vi "TagCreatePixelArray.vi"(5 "Layout":string, 6 "Add Border":bool, 7 "Codes":i64[](array[numeric]), 8 "error in (no error)":errorcluster, 11 "ID":i32) -> (0 "error out":errorcluster, 1 "Alpha":u8[][](array[numeric]), 3 "Pixels":u8[][](array[numeric]))   [LabVIEW 2020, in "feature_detection.lvlib"]
uses:
  feature_detection.lvlib
  TagPixelType.ctl
  <vilib>/Utility/error.llb/Error Cluster From Error Code.vi
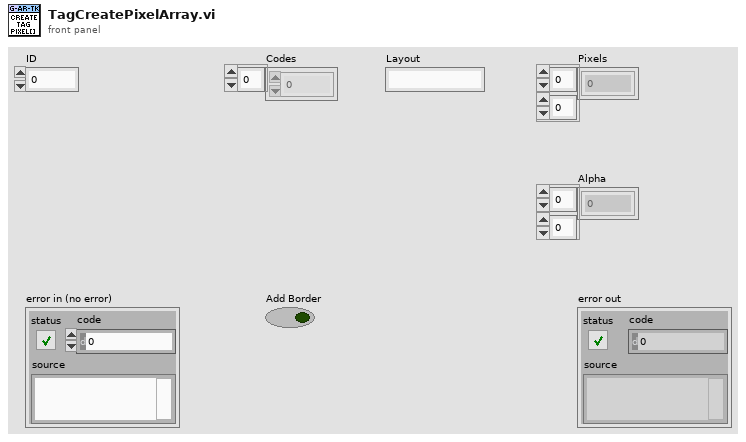
[diagram p1: front panel]
types:
  T1 = typedef "feature_detection.lvlib/TagPixelType.ctl" = enum8{"Black", "White", "Transparent"}
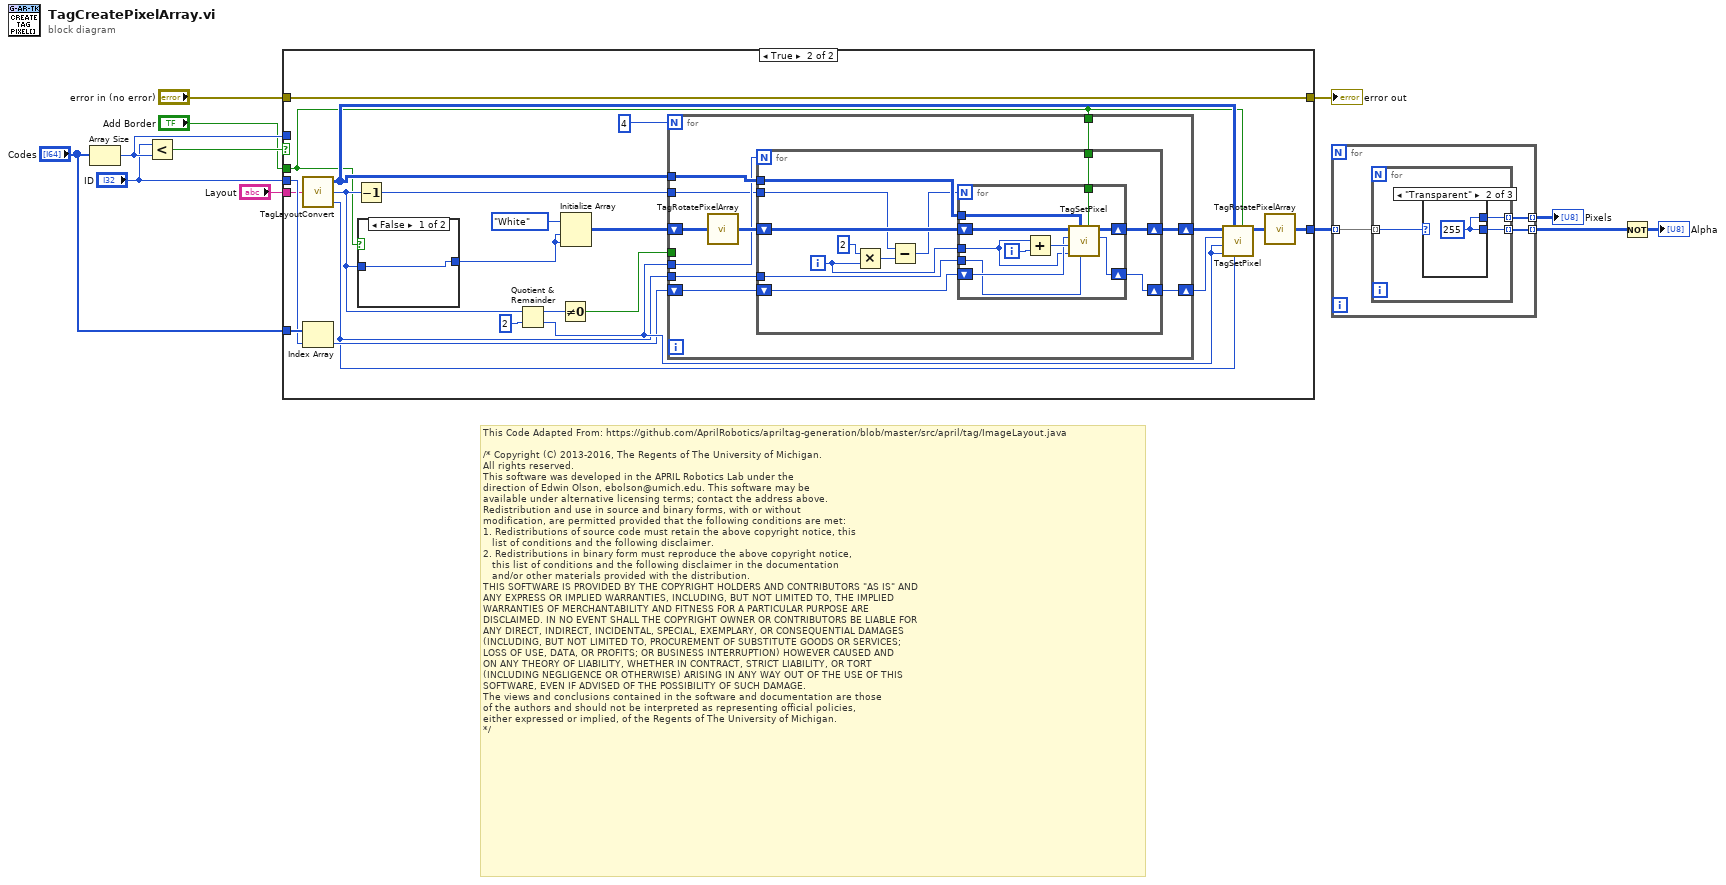
[diagram p0: block diagram]
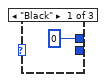
[diagram p2: hidden frame]
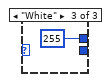
[diagram p3: hidden frame]
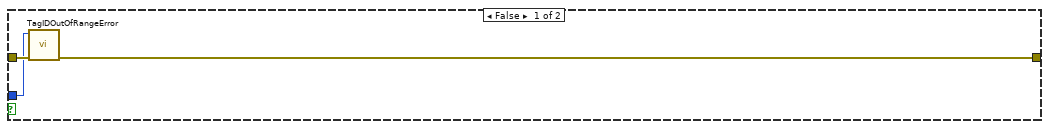
[diagram p4: hidden frame]
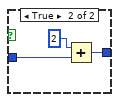
[diagram p5: hidden frame]
diagram:
  # "This Code Adapted From: https://github.com/AprilRobotics/apriltag-generation/blob/master/src/april/tag/ImageLayout.java\n\n/* Copyright (C) 2013-2016, The Regents of The University of Michigan.\nAll rights reserved.\nThis software was developed in the APRIL Robotics Lab under the\ndirection of Edwin Olson, ebolson@umich.edu. This software may be\navailable under alternative licensing terms; contact the address above.\nRedistribution and use in source and binary forms, with or without\nmodification, are permitted provided that the following conditions are met:\n1. Redistributions of source code must retain the above copyright notice, this\n   list of conditions and the following disclaimer.\n2. Redistributions in binary form must reproduce the above copyright notice,\n   this list of conditions and the following disclaimer in the documentation\n   and/or other materials provided with the distribution.\nTHIS SOFTWARE IS PROVIDED BY THE COPYRIGHT HOLDERS AND CONTRIBUTORS \"AS IS\" AND\nANY EXPRESS OR IMPLIED WARRANTIES, INCLUDING, BUT NOT LIMITED TO, THE IMPLIED\nWARRANTIES OF MERCHANTABILITY AND FITNESS FOR A PARTICULAR PURPOSE ARE\nDISCLAIMED. IN NO EVENT SHALL THE COPYRIGHT OWNER OR CONTRIBUTORS BE LIABLE FOR\nANY DIRECT, INDIRECT, INCIDENTAL, SPECIAL, EXEMPLARY, OR CONSEQUENTIAL DAMAGES\n(INCLUDING, BUT NOT LIMITED TO, PROCUREMENT OF SUBSTITUTE GOODS OR SERVICES;\nLOSS OF USE, DATA, OR PROFITS; OR BUSINESS INTERRUPTION) HOWEVER CAUSED AND\nON ANY THEORY OF LIABILITY, WHETHER IN CONTRACT, STRICT LIABILITY, OR TORT\n(INCLUDING NEGLIGENCE OR OTHERWISE) ARISING IN ANY WAY OUT OF THE USE OF THIS\nSOFTWARE, EVEN IF ADVISED OF THE POSSIBILITY OF SUCH DAMAGE.\nThe views and conclusions contained in the software and documentation are those\nof the authors and should not be interpreted as representing official policies,\neither expressed or implied, of the Regents of The University of Michigan.\n*/"
  n1 = Array Size(array="Codes") -> (size(s)=w11:i32)
  n2 = Less?(x="ID", y=w11) -> (x < y?=w8:bool)
  n3 = case shown="True" w8 {
    tunnel: "Codes" -> [_ w37]
    tunnel: "ID" -> [_ w36]
    tunnel: "error in (no error)" -> [w15 w19]
    tunnel: [w14 w19] -> w10
    tunnel: w11 -> [w13 _]
    tunnel: "Layout" -> [_ w23]
    tunnel: [_ w24] -> w5
    tunnel: "Add Border" -> [_ w16]
    frame False {
      n4 = call "TagIDOutOfRangeError.vi"("error in (no error)"=w15, "Tag Family Size"=w13) -> ("error out"=w14:errorcluster)  [unwired: 9 in]
    }
    frame True {
      n5 = call "TagLayoutConvert.vi"("Layout"=w23) -> ("Pixel Map"=w22:u8[][], "Size"=w20:i32, "Number Of Bits"=w21:i32)
      n6 = Index Array(array=w37, index=w36) -> (element=w25:i64)
      n7 = Decrement(x=w20) -> (x-1=w28:i32)
      n8 = case shown="False" w16 {
        tunnel: w20 -> [w38 w41]
        tunnel: [w38 w40] -> w17
        frame False {
        }
        frame True {
          n9 = Add(x=2, y=w41) -> (x+y=w40:i32)
        }
      }
      n10 = Quotient & Remainder(x=w20, y=2) -> (x-y*floor(x/y)=w27:i32, floor(x/y)=w29:i32)
      n11 = Not Equal To 0?(x=w27) -> (x != 0?=w32:bool)
      n12 = Initialize Array(TagPixelType."White", w17, w17) -> (w18:T1[][])
      n13 = for {
        N: 4 -> [_]
        shift-right: [w47] -> w33
        shift-left: w18 -> [w49]
        tunnel: w29 -> [w44]
        tunnel: w28 -> [w43]
        tunnel: w22 -> [w51]
        tunnel: w21 -> [w50]
        tunnel: w32 -> [_]
        shift-right: [w45] -> w35
        shift-left: w25 -> [w46]
        tunnel: w16 -> [w42]
        n14 = call "TagRotatePixelArray.vi"("Pixel Array In"=w49) -> ("Rotated Pixel Array"=w48:T1[][])
        n15 = for {
          N: w44 -> [_]
          tunnel: w51 -> [w63]
          shift-right: [w61] -> w47
          shift-left: w48 -> [w62]
          tunnel: w50 -> [w60]
          shift-right: [w58] -> w45
          shift-left: w46 -> [w59]
          tunnel: w43 -> [w56]
          tunnel: w42 -> [w52]
          i -> [w57]
          n16 = Multiply(x=2, y=w57) -> (x*y=w55:i32)
          n17 = Subtract(x=w56, y=w55) -> (x-y=w53:i32)
          n18 = for {
            N: w53 -> [_]
            tunnel: w57 -> [w66]
            tunnel: w63 -> [w68]
            shift-right: [w72] -> w61
            shift-left: w62 -> [w70]
            tunnel: w60 -> [w65]
            shift-right: [w71] -> w58
            shift-left: w59 -> [w67]
            tunnel: w52 -> [w64]
            i -> [w73]
            n19 = Add(x=w66, y=w73) -> (x+y=w69:i32)
            n20 = call "TagSetPixel.vi"("Add Border"=w64, "Number of Bits"=w65, "Pixel Type Map"=w68, "y"=w66, "x"=w69, "Code in"=w67, "Pixels in"=w70) -> ("Code out"=w71:i64, "Pixels out"=w72:T1[][])  [unwired: 3 in]
          }
        }
      }
      n21 = call "TagSetPixel.vi"("Add Border"=w16, "Number of Bits"=w21, "Pixel Type Map"=w22, "y"=w29, "x"=w29, "Code in"=w35, "Pixels in"=w33) -> ("Pixels out"=w34:T1[][])  [unwired: 3 in, 1 out]
      n22 = call "TagRotatePixelArray.vi"("Pixel Array In"=w34) -> ("Rotated Pixel Array"=w24:T1[][])
    }
  }
  "error out" <- w10
  n23 = for {
    tunnel: w5 -> [w76] mode=indexing
    tunnel: [w75] -> w2 mode=indexing
    tunnel: [w74] -> w4 mode=indexing
    n24 = for {
      tunnel: w76 -> [w79] mode=indexing
      tunnel: [w78] -> w75 mode=indexing
      tunnel: [w77] -> w74 mode=indexing
      n25 = case shown="\"Transparent\"" w79 {
        tunnel: [u8 0 w81 u8 255] -> w78
        tunnel: [_ w81 _] -> w77
        frame "Black" {
        }
        frame "Transparent" {
          w81 = u8 255
        }
        frame "White" {
        }
      }
    }
  }
  "Pixels" <- w2
  n26 = Not(x=w4) -> (.not. x?=→"Alpha":u8[][])
